vi "Refname to String (Queue).vi"(1 "Queue Refname":T1=enum."Drive") -> (0 "Refnum Name":string)   [LabVIEW 2015, in "Sprocket.lvlib"]
uses:
  lib/Sprocket.lvlib
  Refname Enum (Queue).ctl
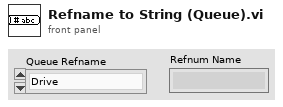
[diagram p1: front panel]
types:
  T1 = typedef "Sprocket.lvlib/Refname Enum (Queue).ctl" = enum16{"Input", "Drive"}
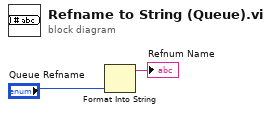
[diagram p0: block diagram]
diagram:
  n1 = Format Into String("Queue Refname") -> (resulting string=→"Refnum Name":string)  [unwired: 3 in, 1 out]
